vi "GetU64.vi"(5 "format string (%_20d)":string="%_20d", 7 "key description":string, 8 "sections":string[](array[string]), 9 "numeric":u64, 11 "info data":string) -> (0 "sections out":string[](array[string]), 1 "found?":bool, 2 "value":u64, 3 "info data out":string)   [LabVIEW 2013, in "infolib.lvlib"]
doc: "Add a new numeric key to Info Data string. If section exists in Info Data string, inserts key into this section."
uses:
  infolib.lvlib
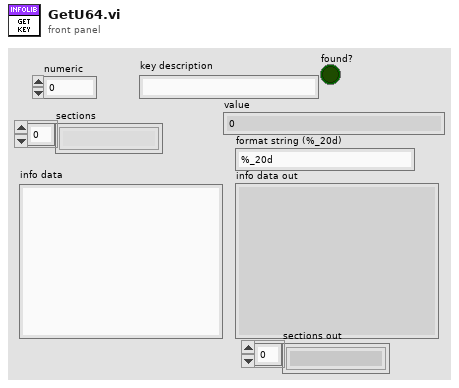
[diagram p1: front panel]
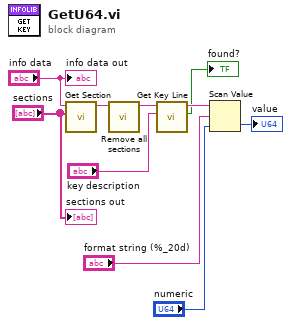
[diagram p0: block diagram]
diagram:
  n1 = call "Get Section.vi"("sections"="sections", "info data"="info data") -> ("section part"=w10:string)  [unwired: 8 in, 1 out]
  n2 = call "Remove all sections.vi"("info data"=w10) -> ("info data out"=w8:string)  [unwired: 10 in]
  n3 = call "Get Key Line.vi"("key description"="key description", "info data"=w8) -> ("found?"=→"found?":bool, "key value"=w4:string)  [unwired: 8 in]
  n4 = Scan Value(string=w4, format string="format string (%_20d)", default (0 dbl)="numeric") -> (value=→"value":u64)  [unwired: 1 out]
  "info data out" <- "info data"
  "sections out" <- "sections"
